vi "Obtain Default Broadcast Events.vi"(8 "error in (no error)":errorcluster) -> (0 "error out":errorcluster, 1 "Update Module Execution Status":refnum<user-event>, 2 "Error Reported":refnum<user-event>, 3 "Status Updated":refnum<user-event>, 4 "System Message":refnum<user-event>, 5 "Module Did Stop":refnum<user-event>)   [LabVIEW 2020, in "StateMachine.lvlib"]
doc: "Encapsulates the module-specific Obtain Broadcast Events for Registration.vi and only returns the default broadcast event references that any HSE DQMH module features. Wrapping the VI allows to programmatically obtain the default event references as the module-specific connector panes are hidden away.\n\n____\nHAMPEL SOFTWARE ENGINEERING v2.6.0 (2023-12-19 10:54)"
uses:
  StateMachine.lvlib
  Status Updated Argument--cluster.ctl
  Error Reported Argument--cluster.ctl
  Stop Argument--cluster.ctl
  Get Module Execution Status Argument--cluster.ctl
  System Message Argument--cluster.ctl
  Libraries/hse-libraries/Source/hse-dqmh/Controls/System Message Source.ctl
  Libraries/hse-libraries/Source/hse-dqmh/hse-dqmh.lvlib
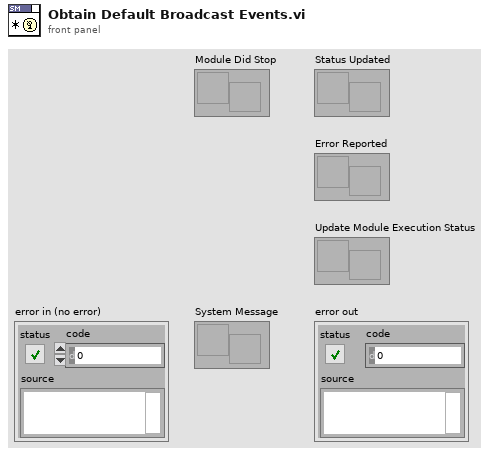
[diagram p1: front panel]
types:
  T1 = typedef "StateMachine.lvlib/Broadcast Events--cluster.ctl" = cluster{"Module Did Init":refnum<user-event>, "Status Updated":refnum<user-event>, "Error Reported":refnum<user-event>, "Module Did Stop":refnum<user-event>, "Update Module Execution Status":refnum<user-event>, "System Message":refnum<user-event>, "DEMO Updated UI State":refnum<user-event>}
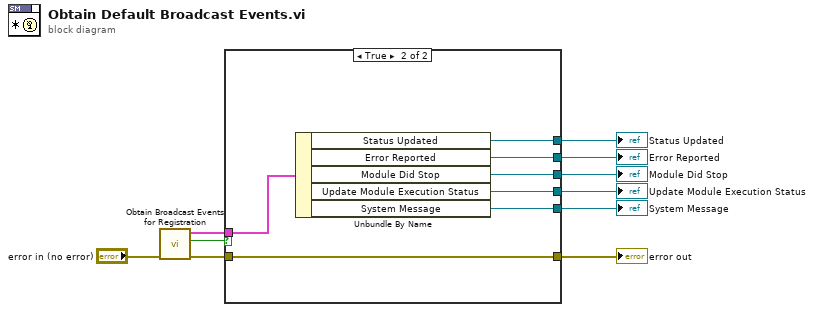
[diagram p0: block diagram]
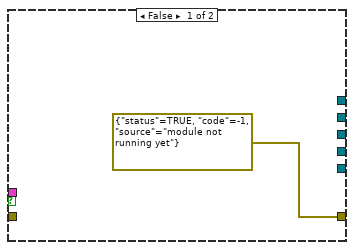
[diagram p2: hidden frame]
diagram:
  n1 = call "Obtain Broadcast Events for Registration.vi"("error in (no error)"="error in (no error)") -> ("error out"=w8:errorcluster, "Already running?"=w9:bool, "StateMachine Broadcast Events"=w6:T1)  [unwired: 8 in]
  n2 = case shown="True" w9 {
    tunnel: [errorcluster {"status"=TRUE, "code"=-1, "source"="module not running yet"} ("error out") w18] -> w7
    tunnel: w8 -> [_ w18]
    tunnel: w6 -> [_ w17]
    tunnel: [_ w16] -> w5
    tunnel: [_ w15] -> w4
    tunnel: [_ w14] -> w3
    tunnel: [_ w13] -> w2
    tunnel: [_ w12] -> w1
    frame False {
    }
    frame True {
      n3 = Unbundle By Name(w17) -> ("Status Updated"=w16:refnum<user-event>, "Error Reported"=w15:refnum<user-event>, "Module Did Stop"=w14:refnum<user-event>, "Update Module Execution Status"=w13:refnum<user-event>, "System Message"=w12:refnum<user-event>)
    }
  }
  "error out" <- w7
  "Status Updated" <- w5
  "Error Reported" <- w4
  "Module Did Stop" <- w3
  "Update Module Execution Status" <- w2
  "System Message" <- w1
